vi "get Description Of Error Code.vi"(8 "error in":errorcluster, 11 "cycloneHandle":u32) -> (0 "error out":errorcluster, 3 "function return":string)   [LabVIEW 2021, in "CycloneControlSDK.lvlib"]
doc: "extern \"C\" char * _cdecl getDescriptionOfErrorCode(uint32_t cycloneHandle, int32_t errorCode);"
uses:
  CycloneControlSDK.lvlib
  CycloneControlSDK_64.dll
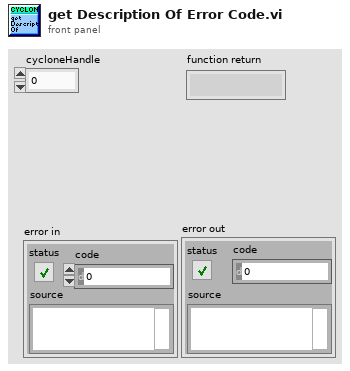
[diagram p1: front panel]
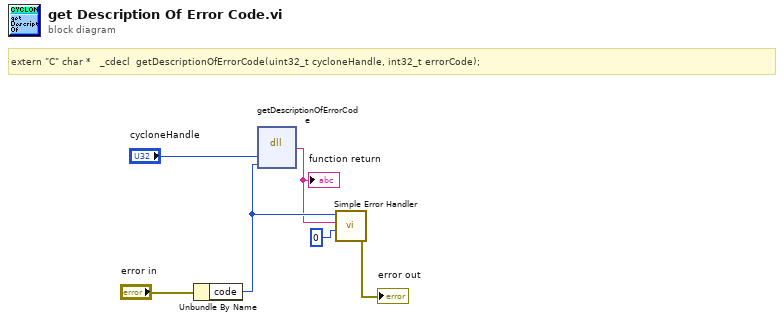
[diagram p0: block diagram]
diagram:
  # "extern \"C\" char *   _cdecl  getDescriptionOfErrorCode(uint32_t cycloneHandle, int32_t errorCode);"
  n1 = Unbundle By Name("error in") -> ("code"=w3:i32)
  n2 = dll-call lib="C:/PEMicro/cyclone/cycloneControl/controlsdk/examples/labview2018/user.lib/CycloneControlSDK/CycloneControlSDK_64.dll" fn="getDescriptionOfErrorCode"("cycloneHandle"="cycloneHandle", "errorCode"=w3) -> ("return type"=w2:string)  [unwired: 5 in, 2 out]
  "function return" <- w2
  n3 = call <vilib>:"Simple Error Handler.vi"("error code (no error:0)"=w3, "error source (\" \")"=w2, "type of dialog (OK msg:1)"=0) -> ("error out"=→"error out":errorcluster)  [unwired: 2 in, 4 out]
